vi "PDIPM_new_X.vi"(8 "alpha":dbl=0.01, 9 "beta":dbl=0.5, 10 "m_mu":dbl=5.0, 11 "convergence\ncriterion":dbl=5e-06) -> (2 "duality gap":dbl, 3 "Q_num":dbl[](array[numeric]))   [LabVIEW 2019]
uses:
  <vilib>/Analysis/_algsub.llb/Vector Norm Type.ctl
  <vilib>/Analysis/_algsub.llb/Real Vector Norm.vi
  <vilib>/Analysis/Matrix/Numeric/Conversions/Array To Matrix - RA2.vi
  <vilib>/Analysis/baseanly.llb/Real Inverse Matrix.vi
  <vilib>/Analysis/Matrix/Numeric/Conversions/Array To Matrix - RA.vi
  <vilib>/Analysis/Matrix/Numeric/Multiply/Multiply - RM,R.vi
  <vilib>/Analysis/Matrix/Numeric/Multiply/Multiply - RM,RM.vi
  <vilib>/Analysis/Matrix/NI_Matrix.lvlib
  <vilib>/Analysis/NI_AALBase.lvlib
  <vilib>/Analysis/NI_AALPro.lvlib
panel:
  out "q for\nMATLAB":string
  out "Timing\nPDIPM":u32
  out "Timing\nread data":u32
  out "r(xp, lmdp) feasible":bool
  out "wrong\nLine search":bool
  out "wrong\nKKT inverse":bool
  out "outer loop":i32
  out "inner loop":i32
  out "lmd_opt feasible":bool[](array[boolean])
  out "lmd_opt":dbl[](array[numeric])
  out "fi":dbl[](array[numeric])
  out "fi_opt feasible":bool[](array[boolean])
  # "Parameter setting"
  # "Backtracking Line Search"
  # "Result"
  # "ERROR"
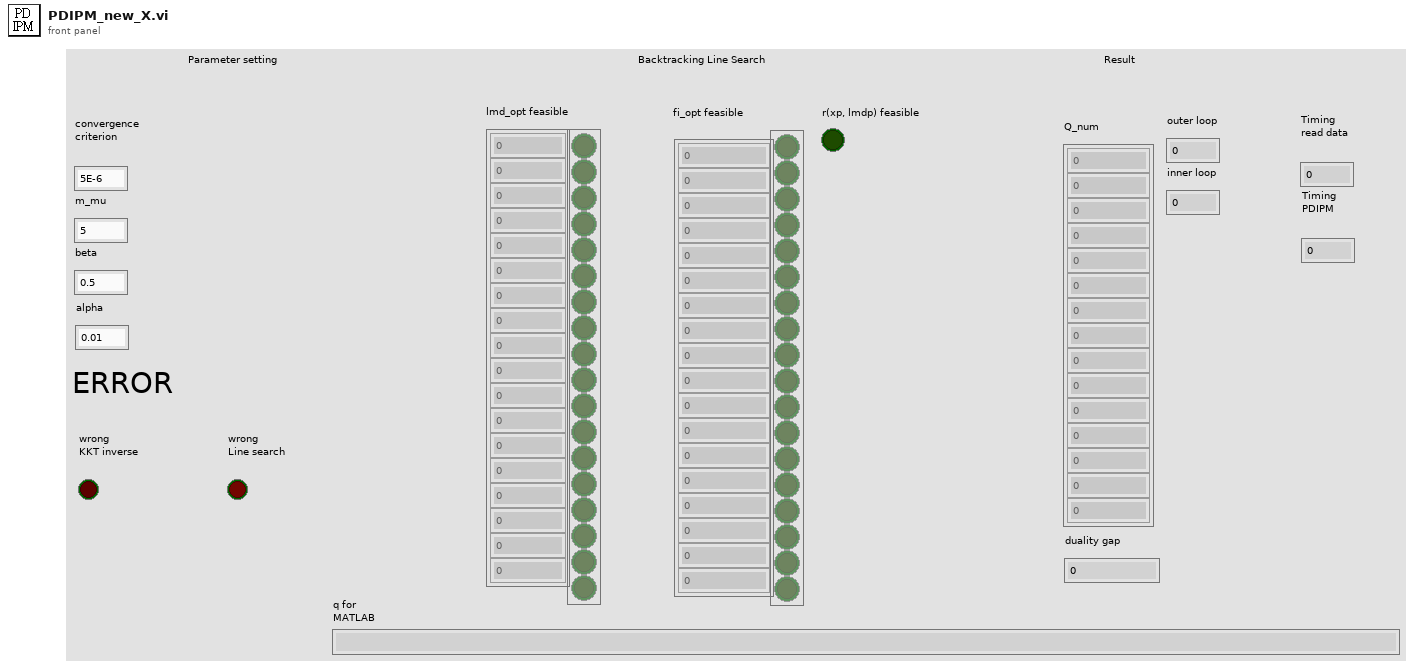
[diagram p1: front panel]
types:
  T1 = cluster{"w0":dbl, "contraints":cluster{"beta":dbl[], "gamma":dbl, "OmegaChain":dbl[], "weight":dbl}[], "Nc":i32}
  T2 = cluster{"weight":dbl, "object":cluster{"beta":dbl[], "gamma":dbl, "OmegaChain":dbl[][]}}
  T3 = typedef "NI_Matrix.lvlib/RealMatrix.ctl" = dbl[][]
  T4 = typedef "NI_AALPro.lvlib/Vector Norm Type.ctl" = u16
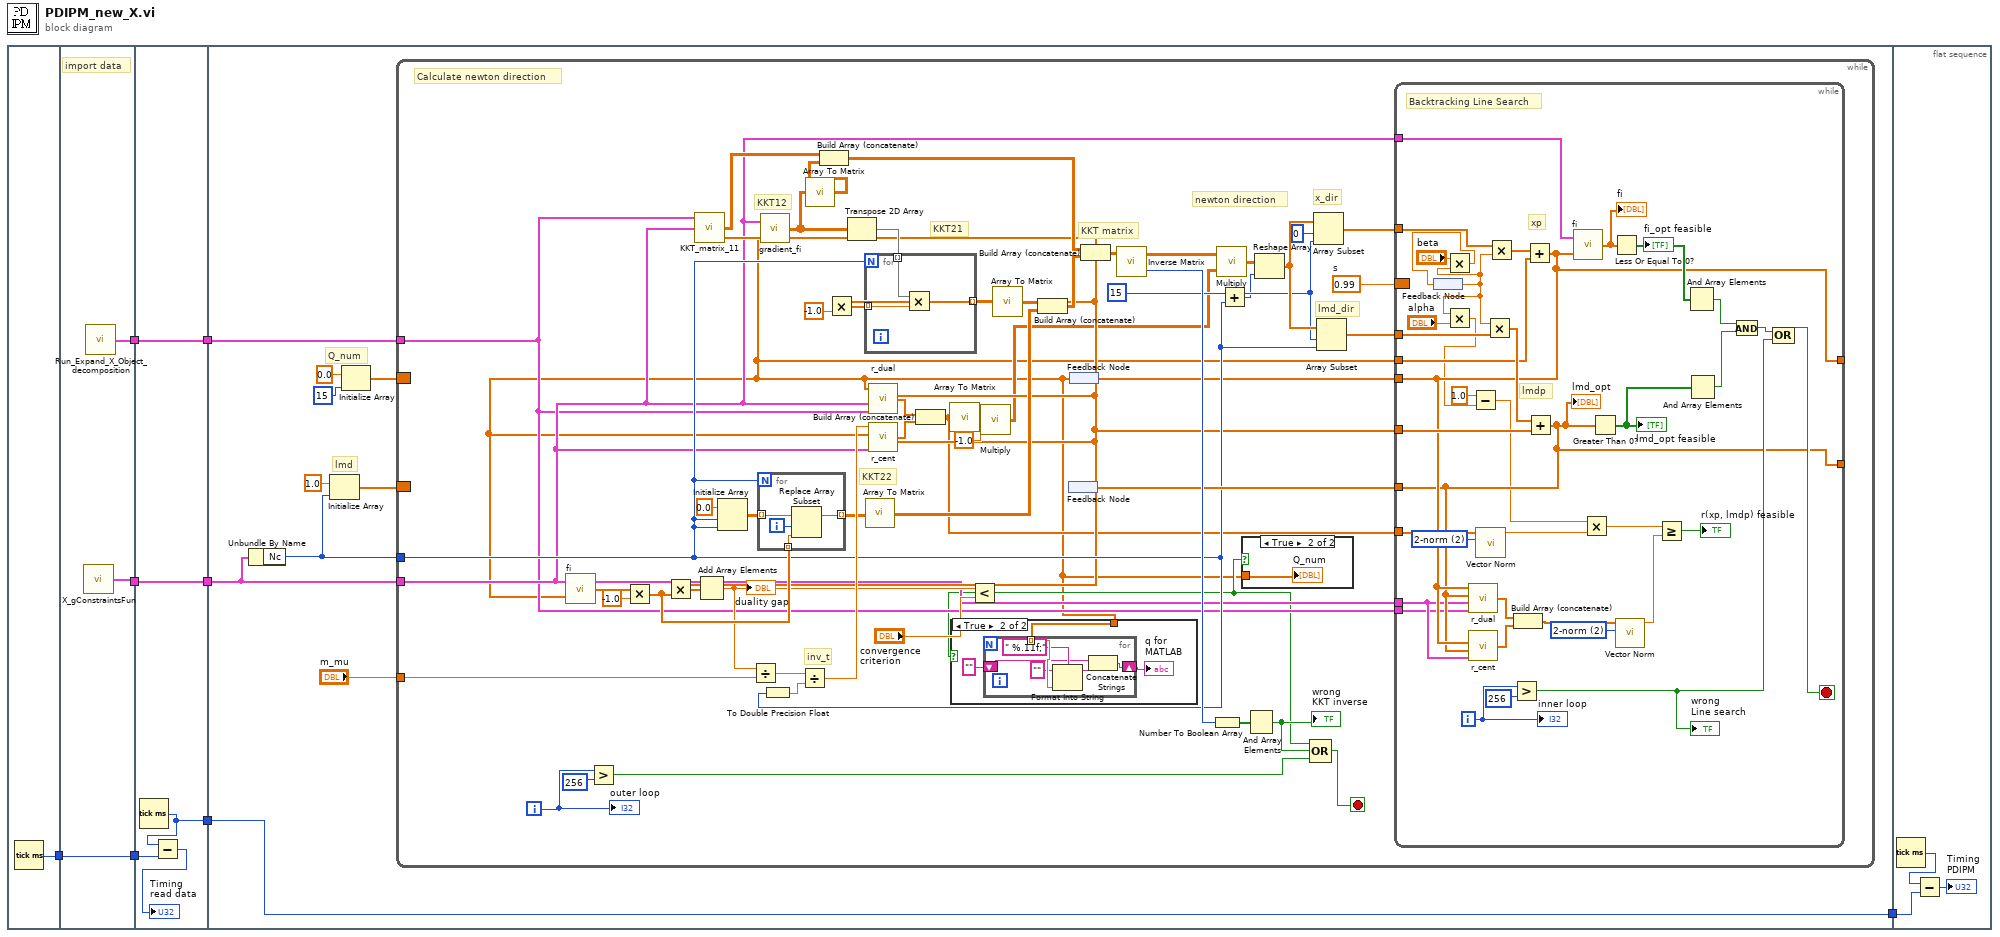
[diagram p0: block diagram]
diagram:
  n1 = flat-sequence {
    tunnel: [w9] -> w4
    tunnel: [w11] -> w7
    tunnel: [w12] -> w5
    tunnel: w4 -> [w12]
    tunnel: [w10] -> w1
    tunnel: [w17] -> w8
    tunnel: w7 -> [w16]
    tunnel: [w16] -> w6
    tunnel: w5 -> [w15]
    tunnel: [w13] -> w2
    tunnel: w1 -> [w17]
    tunnel: w8 -> [w21]
    tunnel: w6 -> [w26]
    tunnel: [w18] -> w3
    tunnel: w2 -> [w18]
    tunnel: w3 -> [w139]
    frame #0 {
      n2 = Tick Count (ms)() -> (millisecond timer value=w9:u32)
    }
    frame #1 {
      # "import data"
      n3 = call "X_gConstraintsFun.vi"() -> ("constraints cluster"=w10:T1)
      n4 = call "Run_Expand_X_Object_decomposition.vi"() -> ("object cluster"=w11:T2)
    }
    frame #2 {
      n5 = Tick Count (ms)() -> (millisecond timer value=w13:u32)
      n6 = Subtract(x=w13, y=w15) -> (x-y=→"Timing\nread data":u32)
    }
    frame #3 {
      # "lmd"
      # "Q_num"
      n7 = Unbundle By Name(w21) -> ("Nc"=w20:i32)
      n8 = Initialize Array(1.0 ("element"), w20) -> (w19:dbl[])
      n9 = Initialize Array(0.0 ("element"), 15 ("dimension size")) -> (w23:dbl[])
      n10 = while {
        tunnel: w21 -> [w35]
        tunnel: "m_mu" -> [w80]
        tunnel: w26 -> [w34]
        border: w23 -> [_]
        tunnel: w20 -> [w41]
        border: w19 -> [_]
        i -> [w57]
        stop <- w52 stop-if-true
        w59 = 0.99  # s
        w44 = 15 ("index")
        # "Calculate newton direction"
        # "KKT22"
        # "newton direction"
        # "lmd_dir"
        # "x_dir"
        # "KKT matrix"
        # "KKT21"
        # "KKT12"
        # "inv_t"
        n11 = Greater?(x=w57, y=256) -> (0:w55:bool)
        n12 = Initialize Array(0.0 ("element"), w41, w41) -> (w73:dbl[][])
        n13 = To Double Precision Float(number=w41) -> (double precision float=w78:dbl)
        n14 = feedback #1() -> (w39:dbl[])
        n15 = call "KKT_matrix_11.vi"("lmd_input"=w39, "constraints cluster"=w35, "Object cluster"=w34) -> ("KKT_matrix_11"=w71:T3)
        n16 = Multiply(x=w39, y=-1.0) -> (x*y=w49:dbl[])
        n17 = feedback #2() -> (w28:dbl[])
        n18 = call "fi.vi"("q_input"=w28, "constraints cluster"=w35) -> ("fi"=w46:dbl[])
        n19 = Multiply(x=w46, y=-1.0) -> (x*y=w72:dbl[])
        n20 = Multiply(x=w39, y=w72) -> (x*y=w81:dbl[])
        n21 = Add Array Elements(numeric array=w81) -> (sum=w50:dbl)
        "duality gap" <- w50
        n22 = Divide(x=w50, y=w80) -> (x/y=w79:dbl)
        n23 = for {
          N: w41 -> [_]
          tunnel: w73 -> [w134] mode=indexing
          tunnel: w72 -> [w132] mode=indexing
          tunnel: [w131] -> w68 mode=indexing
          i -> [w133]
          n24 = Replace Array Subset(array=w134, new element=w132, index=w133) -> (w131:dbl[])
        }
        n25 = call "gradient_fi.vi"("q_input"=w28, "constraints cluster"=w35) -> ("gradient of fi"=w48:dbl[][])
        n26 = Divide(x=w79, y=w78) -> (x/y=w77:dbl)
        n27 = call-poly <vilib>:"Array To Matrix.vi"("Real 2D Array"=w48) -> ("Real Matrix"=w38:T3)
        n28 = Build Array (concatenate)(w71, w38) -> (w66:T3)
        n29 = Transpose 2D Array(2D array=w48) -> (transposed array=w47:dbl[][])
        n30 = for {
          N: w41 -> [_]
          tunnel: w49 -> [w136] mode=indexing
          tunnel: w47 -> [w137] mode=indexing
          tunnel: [w135] -> w70 mode=indexing
          n31 = Multiply(x=w137, y=w136) -> (x*y=w135:dbl[])
        }
        n32 = call-poly <vilib>:"Array To Matrix.vi"("Real 2D Array"=w68) -> ("Real Matrix"=w67:T3)
        n33 = call "r_dual.vi"("object cluster"=w34, "constraints cluster"=w35, "lmd_input"=w39, "q_input"=w28) -> ("dual residual"=w33:dbl[])
        n34 = call "r_cent.vi"("constraints cluster"=w35, "lmd_input"=w39, "q_input"=w28, "inv_t"=w77) -> ("central residual"=w76:dbl[])
        n35 = Build Array (concatenate)(w33, w76) -> (w31:dbl[])
        n36 = call-poly <vilib>:"Array To Matrix.vi"("Real 1D Array"=w31) -> ("Real Matrix (Column Vector)"=w32:T3)
        n37 = Less?(x=w50, y="convergence\ncriterion") -> (x < y?=w29:bool)
        n38 = case shown="True" w29 {
          tunnel: w28 -> [_ w86]
          frame False {
          }
          frame True {
            n39 = for {
              tunnel: w86 -> [w92] mode=indexing
              shift-right: [w88] -> w84
              shift-left: "" ("initial string") -> [w89]
              n40 = Format Into String(format string=" %.11f;", initial string="", w92) -> (resulting string=w90:string)  [unwired: 1 in, 1 out]
              n41 = Concatenate Strings(w89, w90) -> (w88:string)
            }
            "q for\nMATLAB" <- w84
          }
        }
        n42 = call-poly <vilib>:"Multiply.vi"("Real Scalar c"=-1.0, "Real Matrix A"=w32) -> ("A * c"=w37:T3)
        n43 = call-poly <vilib>:"Array To Matrix.vi"("Real 2D Array"=w70) -> ("Real Matrix"=w69:T3)
        n44 = Build Array (concatenate)(w69, w67) -> (w65:T3)
        n45 = Build Array (concatenate)(w66, w65) -> (w45:T3)
        n46 = call-poly <vilib>:"Inverse Matrix.vi"("Input Matrix"=w45) -> ("error"=w56:i32, "Inverse Matrix"=w63:T3)  [unwired: 1 in]
        n47 = Number To Boolean Array(number=w56) -> (Boolean array=w54:bool[])
        n48 = call-poly <vilib>:"Multiply.vi"("Real Matrix B"=w37, "Real Matrix A"=w63) -> ("A * B"=w62:T3)
        n49 = Add(x=w44, y=w41) -> (x+y=w36:i32)
        n50 = case shown="True" w29 {
          tunnel: w28 -> [_ w83]
          frame False {
          }
          frame True {
            "Q_num" <- w83
          }
        }
        n51 = And Array Elements(Boolean array=w54) -> (logical AND=w53:bool)
        "wrong\nKKT inverse" <- w53
        n52 = Reshape Array(w62, w36) -> (w60:dbl[])
        n53 = Compound Arithmetic op=OR(w29, w53, w55) -> (w52:bool)
        n54 = Array Subset(array=w60, index=0, length=w44) -> (w43:dbl[])
        n55 = Array Subset(array=w60, index=w44, length=w41) -> (w40:dbl[])
        n56 = while {
          tunnel: w43 -> [w114]
          tunnel: w40 -> [w115]
          tunnel: w35 -> [w129]
          border: w59 -> [_]
          tunnel: [w109] -> w42
          tunnel: [w110] -> w30
          tunnel: w28 -> [w113]
          tunnel: [w110] -> _
          tunnel: w39 -> [w112]
          tunnel: [w109] -> _
          tunnel: w35 -> [w108]
          tunnel: w34 -> [w107]
          tunnel: w31 -> [w102]
          i -> [w122]
          stop <- w116 stop-if-true
          w104 = T4 2 items=["1-norm"=1, "2-norm"=2, "Inf-norm"=3, "-Inf-norm"=4, "User Defined"=5] ("norm type")
          w111 = T4 2 items=["1-norm"=1, "2-norm"=2, "Inf-norm"=3, "-Inf-norm"=4, "User Defined"=5] ("norm type")
          # "lmdp"
          # "xp"
          # "Backtracking Line Search"
          n57 = feedback #3() -> (w100:dbl)
          n58 = Multiply(x="beta", y=w100) -> (x*y=w117:dbl)
          n59 = feedback-in #3(w117) -> ()
          n60 = Multiply(x=w100, y="alpha") -> (x*y=w99:dbl)
          n61 = Subtract(x=1.0, y=w99) -> (x-y=w97:dbl)
          n62 = call-poly <vilib>:"Vector Norm.vi"("norm type"=w111, "Input Vector"=w102) -> ("norm"=w96:dbl)  [unwired: 8 in, 1 out]
          n63 = Multiply ("Multiply.vi")(x=w100, y=w115) -> (x*y=w119:dbl[])
          n64 = Multiply ("Multiply.vi")(x=w114, y=w100) -> (x*y=w130:dbl[])
          n65 = Greater?(x=w122, y=256) -> (0:w120:bool)
          "wrong\nLine search" <- w120
          n66 = Add(x=w130, y=w113) -> (x+y=w110:dbl[])
          n67 = Add(x=w119, y=w112) -> (x+y=w109:dbl[])
          "lmd_opt" <- w109
          n68 = call "r_dual.vi"("object cluster"=w107, "constraints cluster"=w108, "lmd_input"=w109, "q_input"=w110) -> ("dual residual"=w106:dbl[])
          n69 = call "r_cent.vi"("constraints cluster"=w108, "lmd_input"=w109, "q_input"=w110) -> ("central residual"=w105:dbl[])  [unwired: 1 in]
          n70 = Build Array (concatenate)(w106, w105) -> (w103:dbl[])
          n71 = call "fi.vi"("q_input"=w110, "constraints cluster"=w129) -> ("fi"=w128:dbl[])
          "fi" <- w128
          n72 = Multiply(x=w97, y=w96) -> (x*y=w95:dbl)
          n73 = Greater Than 0?(x=w109) -> (x > 0?=w126:bool[])
          "lmd_opt feasible" <- w126
          n74 = Less Or Equal To 0?(x=w128) -> (x <= 0?=w127:bool[])
          "fi_opt feasible" <- w127
          n75 = call-poly <vilib>:"Vector Norm.vi"("norm type"=w104, "Input Vector"=w103) -> ("norm"=w94:dbl)  [unwired: 8 in, 1 out]
          n76 = Greater Or Equal?(x=w95, y=w94) -> (x >= y?=→"r(xp, lmdp) feasible":bool)
          n77 = And Array Elements(Boolean array=w127) -> (logical AND=w125:bool)
          n78 = And Array Elements(Boolean array=w126) -> (logical AND=w124:bool)
          n79 = Compound Arithmetic op=AND(w125, w124) -> (w123:bool)
          n80 = Compound Arithmetic op=OR(w123, w120) -> (w116:bool)
          "inner loop" <- w122
        }
        n81 = feedback-in #1(w42) -> ()
        n82 = feedback-in #2(w30) -> ()
        "outer loop" <- w57
      }
    }
    frame #4 {
      n83 = Tick Count (ms)() -> (millisecond timer value=w140:u32)
      n84 = Subtract(x=w140, y=w139) -> (x-y=→"Timing\nPDIPM":u32)
    }
  }
